vi "QueueGetTestCaseID.vi"() -> (3 "test case ID":string)   [LabVIEW 2018]
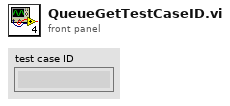
[diagram p1: front panel]
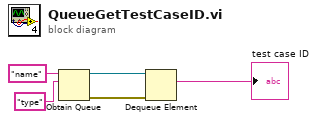
[diagram p0: block diagram]
diagram:
  n1 = Obtain Queue(name (unnamed)="name", element data type="type" ("name (unnamed)")) -> (queue out=w3:refnum<queue>, error out=w2:errorcluster)  [unwired: 3 in, 1 out]
  n2 = Dequeue Element(queue=w3, error in (no error)=w2) -> (element=→"test case ID":string)  [unwired: 1 in, 3 out]
